vi "Blob Selection.vi"(11 "Acceptable Blobs + Scores":T1[](array[typedef])) -> (2 "Acceptable Left Blobs":T1[](array[typedef]), 3 "Acceptable Right Blobs":T1[](array[typedef]))   [LabVIEW 2014]
uses:
  target type.ctl
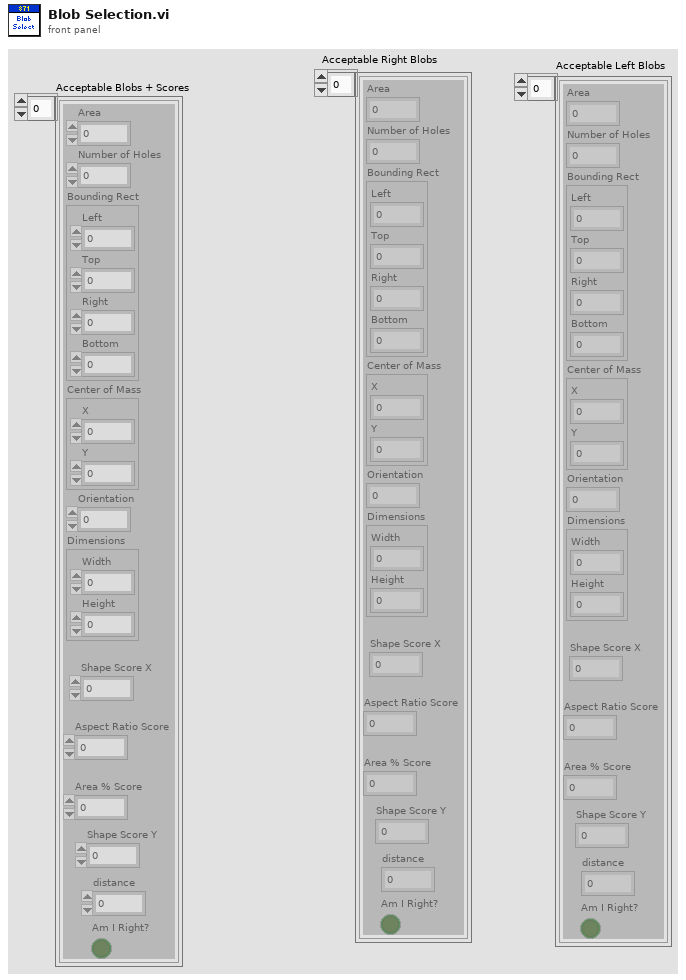
[diagram p1: front panel]
types:
  T1 = typedef "target type.ctl" = cluster{"Area":dbl, "Number of Holes":dbl, "Bounding Rect":cluster{"Left":dbl, "Top":dbl, "Right":dbl, "Bottom":dbl}, "Center of Mass":cluster{"X":dbl, "Y":dbl}, "Orientation":dbl, "Dimensions":cluster{"Width":dbl, "Height":dbl}, "Shape Score X":dbl, "Aspect Ratio Score":dbl, "Area % Score":dbl, "Shape Score Y":dbl, "Am I Right?":bool, "distance":dbl}
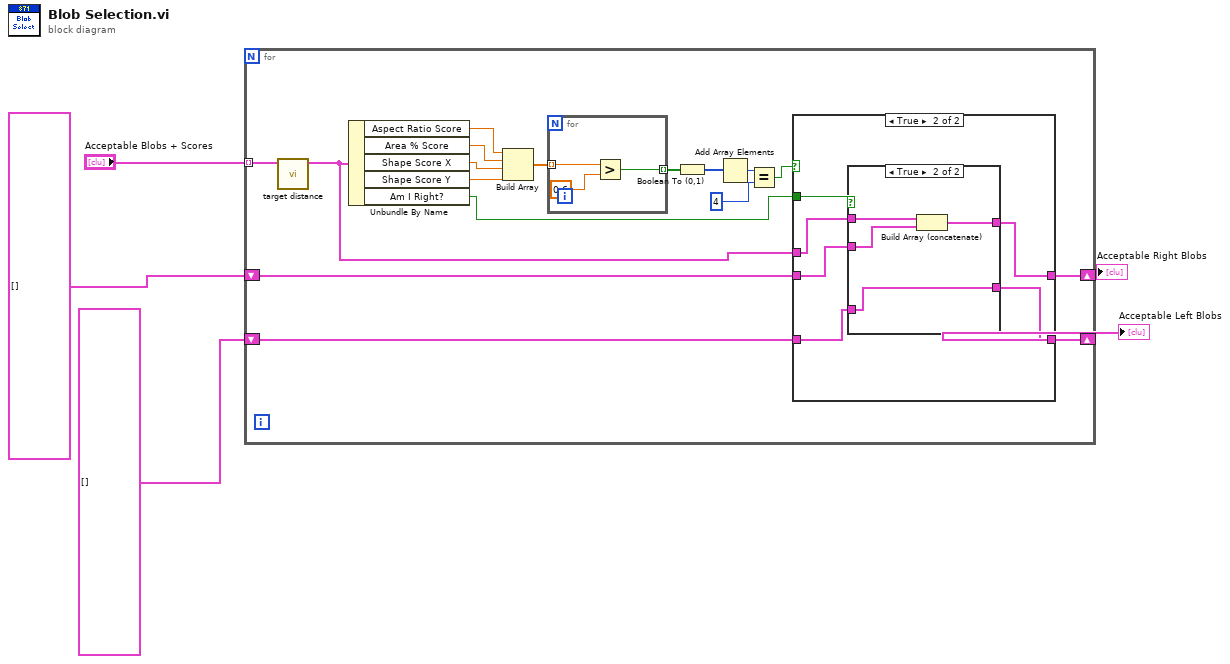
[diagram p0: block diagram]
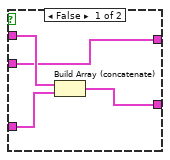
[diagram p3: hidden frame]
diagram:
  n1 = for {
    tunnel: "Acceptable Blobs + Scores" -> [w7] mode=indexing
    shift-right: [w12] -> w3
    shift-left: T1[] [] ("Acceptable Blobs + Scores 2") -> [w11]
    shift-right: [w9] -> w1
    shift-left: T1[] [] ("Acceptable Blobs + Scores 2") -> [w10]
    n2 = call "target distance.vi"("Blobs"=w7) -> ("Blobs + distance"=w6:T1)  [unwired: 10 in]
    n3 = Unbundle By Name(w6) -> ("Aspect Ratio Score"=w22:dbl, "Area % Score"=w21:dbl, "Shape Score X"=w20:dbl, "Shape Score Y"=w19:dbl, "Am I Right?"=w8:bool)
    n4 = Build Array(w22, w21, w20, w19) -> (w18:dbl[])
    n5 = for {
      tunnel: w18 -> [w41] mode=indexing
      tunnel: [w39] -> w17 mode=indexing
      n6 = Greater?(x=w41, y=0.6) -> (0:w39:bool)
    }
    n7 = Boolean To (0,1)(Boolean=w17) -> (0, 1=w16:i16[])
    n8 = Add Array Elements(numeric array=w16) -> (sum=w15:i16)
    n9 = Equal?(x=w15, y=4) -> (x = y?=w14:bool)
    n10 = case shown="True" w14 {
      tunnel: w6 -> [_ w29]
      tunnel: [w24 w30] -> w12
      tunnel: w11 -> [w24 w27]
      tunnel: w10 -> [w23 w26]
      tunnel: [w23 w25] -> w9
      tunnel: w8 -> [_ w28]
      frame False {
      }
      frame True {
        n11 = case shown="True" w28 {
          tunnel: [w31 w36] -> w30
          tunnel: w29 -> [w34 w38]
          tunnel: w27 -> [w31 w37]
          tunnel: w26 -> [w33 w35]
          tunnel: [w32 w35] -> w25
          frame False {
            n12 = Build Array (concatenate)(w34, w33) -> (w32:T1[])
          }
          frame True {
            n13 = Build Array (concatenate)(w38, w37) -> (w36:T1[])
          }
        }
      }
    }
  }
  "Acceptable Right Blobs" <- w3
  "Acceptable Left Blobs" <- w1
